vi "Aggiorna colori caselle.vi"(7 "id":i32, 10 "Letture inverter":T1, 11 "Test settings":refnum<vi>) -> ()   [LabVIEW 2019]
uses:
  Letture inverter.ctl
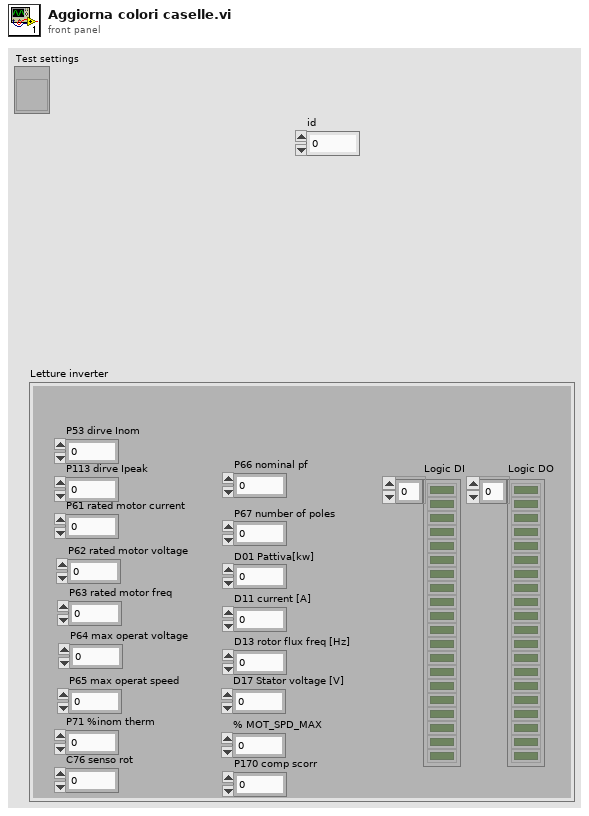
[diagram p1: front panel]
types:
  T1 = typedef "Letture inverter.ctl" = cluster{"P61 rated motor current":dbl, "P62 rated motor voltage":dbl, "P63 rated motor freq":dbl, "P64 max operat voltage":dbl, "P65 max operat speed":dbl, "P66 nominal pf":dbl, "P67 number of poles":dbl, "D01 Pattiva[kw]":dbl, "D11 current [A]":dbl, "D13 rotor flux freq [Hz]":dbl, "D17 Stator voltage [V]":dbl, "% MOT_SPD_MAX":dbl, "Logic DI":bool[], "Logic DO":bool[], "P71 %inom therm":dbl, "P53 dirve Inom":dbl, "P113 dirve Ipeak":dbl, "C76 senso rot":dbl, "P170 comp scorr":dbl}
  T2 = typedef "Parametri inverter.ctl" = cluster{"Vn [V]":dbl, "Fn [Hz]":dbl, "CosFi":dbl, "Imax [%Inom]":dbl, "#poles":dbl, "Inom [A]":dbl, "Senso rotazione":enum16{"CW", "CCW"}, "RPM nom":dbl, "Fmax[Hz]":dbl}
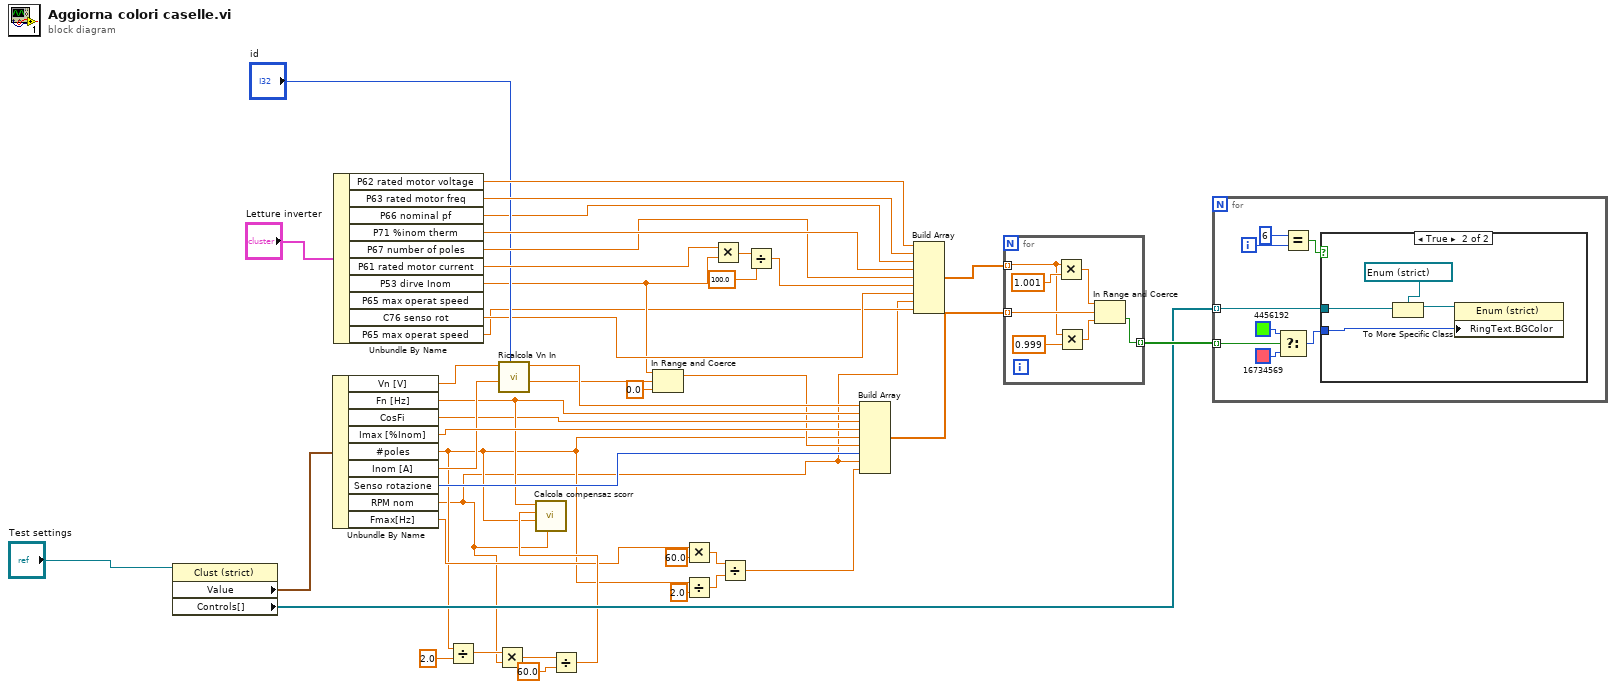
[diagram p0: block diagram]
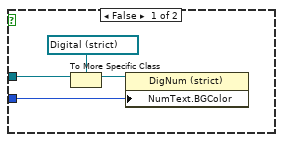
[diagram p2: hidden frame]
diagram:
  n1 = property class="Clust (strict)"(reference="Test settings") -> ("Value"=w28:T2, "Controls[]"=w33:refnum<vi>[])  [unwired: 1 in, 2 out]
  n2 = Unbundle By Name(w28) -> ("Vn [V]"=w32:dbl, "Fn [Hz]"=w23:dbl, "CosFi"=w22:dbl, "Imax [%Inom]"=w35:dbl, "#poles"=w3:dbl, "Inom [A]"=w30:dbl, "Senso rotazione"=w24:enum16{"CW", "CCW"}, "RPM nom"=w1:dbl, "Fmax[Hz]"=w4:dbl)
  n3 = Unbundle By Name("Letture inverter") -> ("P62 rated motor voltage"=w39:dbl, "P63 rated motor freq"=w38:dbl, "P66 nominal pf"=w16:dbl, "P71 %inom therm"=w37:dbl, "P67 number of poles"=w36:dbl, "P61 rated motor current"=w41:dbl, "P53 dirve Inom"=w12:dbl, "C76 senso rot"=w25:dbl, "P65 max operat speed"=w10:dbl)  [unwired: 1 out]
  n4 = Divide(x=w3, y=2.0) -> (x/y=w20:dbl)
  n5 = Multiply(x=w20, y=w1) -> (x*y=w19:dbl)
  n6 = call "Ricalcola Vn In.vi"("id"="id", "In [A]"=w30, "Vn [V]"=w32) -> ("In out"=w14:dbl, "Vn out"=w31:dbl)  [unwired: 7 in]
  n7 = Divide(x=w19, y=60.0) -> (x/y=w17:dbl)
  n8 = call "Calcola compensaz scorr.vi"("RPM nom"=w1, "#poles"=w3, "Fmax [Hz]"=w17, "Fn [Hz]"=w23) -> ()  [unwired: 7 in, 1 out]
  n9 = In Range and Coerce(upper limit=w12, x=w14, lower limit=0.0) -> (coerced(x)=w11:dbl)  [unwired: 1 out]
  n10 = Multiply(x=w4, y=60.0) -> (x*y=w6:dbl)
  n11 = Divide(x=w3, y=2.0) -> (x/y=w8:dbl)
  n12 = Multiply(x=w41, y=w12) -> (x*y=w42:dbl)
  n13 = Divide(x=w6, y=w8) -> (x/y=w2:dbl)
  n14 = Divide(x=w42, y=100.0) -> (x/y=w15:dbl)
  n15 = Build Array(w31, w23, w22, w35, w3, w11, w24, w1, w2) -> (w40:dbl[])
  n16 = Build Array(w39, w38, w16, w37, w36, w15, w25, w1, w10) -> (w26:dbl[])
  n17 = for {
    tunnel: w26 -> [w47] mode=indexing
    tunnel: w40 -> [w50] mode=indexing
    tunnel: [w44] -> w34 mode=indexing
    n18 = Multiply(x=w47, y=1.001) -> (x*y=w48:dbl)
    n19 = Multiply(x=w47, y=0.999) -> (x*y=w45:dbl)
    n20 = In Range and Coerce(upper limit=w48, x=w50, lower limit=w45) -> (In Range?=w44:bool)  [unwired: 1 out]
  }
  n21 = for {
    tunnel: w33 -> [w58] mode=indexing
    tunnel: w34 -> [w57] mode=indexing
    i -> [w53]
    n22 = Select(t=u32 4456192, s=w57, f=u32 16734569) -> (s? t:f=w54:u32)
    n23 = Equal?(x=6, y=w53) -> (x = y?=w51:bool)
    n24 = case shown="True" w51 {
      tunnel: w58 -> [w62 w65]
      tunnel: w54 -> [w61 w64]
      frame False {
        n25 = To More Specific Class(target class=refnum<vi> refnum ("Vn [V]"), reference=w62) -> (specific class reference=w60:refnum<vi>)  [unwired: 1 in, 1 out]
        n26 = property class="DigNum (strict)"(reference=w60, "NumText.BGColor"=w61) -> ()  [unwired: 1 in, 2 out]
      }
      frame True {
        n27 = To More Specific Class(target class=refnum<vi> refnum ("Senso rotazione"), reference=w65) -> (specific class reference=w66:refnum<vi>)  [unwired: 1 in, 1 out]
        n28 = property class="Enum (strict)"(reference=w66, "RingText.BGColor"=w64) -> ()  [unwired: 1 in, 2 out]
      }
    }
  }
